vi "changecolor.vi"(8 "error in (no error)":errorcluster, 9 "Numeric":i32, 10 "Boolean":bool, 11 "MulticolumnListbox in":refnum<vi>) -> (0 "error out":errorcluster, 3 "MulticolumnListbox out":refnum<vi>)   [LabVIEW 2022 SP3]
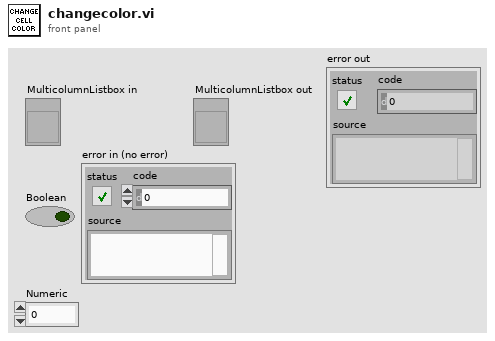
[diagram p1: front panel]
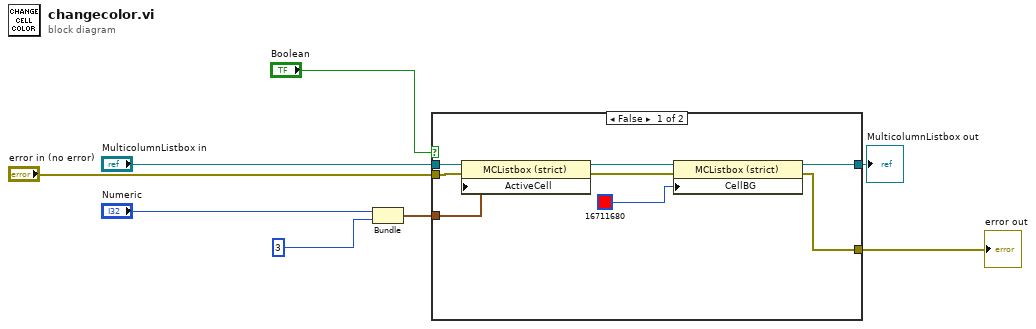
[diagram p0: block diagram]
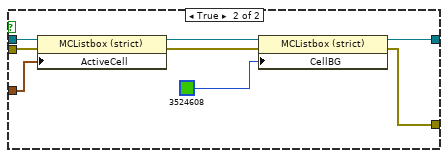
[diagram p2: hidden frame]
diagram:
  n1 = Bundle("Numeric"="Numeric", "Column"=3) -> (w6:cluster{"Numeric":i32, "Column":i32})  [unwired: 1 in]
  n2 = case shown="False" "Boolean" {
    tunnel: "MulticolumnListbox in" -> [w15 w24]
    tunnel: [w13 w22] -> w5
    tunnel: w6 -> [w14 w21]
    tunnel: [w11 w20] -> w2
    tunnel: "error in (no error)" -> [w10 w18]
    frame False {
      n3 = property class="MCListbox (strict)"(reference=w15, error in=w10, "ActiveCell"=w14) -> (reference out=w16:refnum<vi>, error out=w12:errorcluster)
      n4 = property class="MCListbox (strict)"(reference=w16, error in=w12, "CellBG"=u32 16711680) -> (reference out=w13:refnum<vi>, error out=w11:errorcluster)
    }
    frame True {
      n5 = property class="MCListbox (strict)"(reference=w24, error in=w18, "ActiveCell"=w21) -> (reference out=w23:refnum<vi>, error out=w19:errorcluster)
      n6 = property class="MCListbox (strict)"(reference=w23, error in=w19, "CellBG"=u32 3524608) -> (reference out=w22:refnum<vi>, error out=w20:errorcluster)
    }
  }
  "MulticolumnListbox out" <- w5
  "error out" <- w2
